vi "User Actor Core Init.vi"(0 "Module in":refnum<class "Module.lvclass">, 11 "Error in":errorcluster caption="Error in (no error)") -> (4 "Module out":refnum<class "Module.lvclass">, 15 "Error out":errorcluster)   [LabVIEW 2019, in "GP Module.lvlib" / "Module.lvclass"]
doc: "Initialize custom <B>Actor</B> resources. Typical actions:\n\n- Open/create own references.\n- Initialize SW resources.\n- Initialize HW resources.\n- Register additional user events. Beware that external user events are a potential for message racing as those are extra communication channels into <B>Actor</B> that does not follow the message order imposed by the Actor communication tree. If possible convert user event based APIs into message based APIs.\n\n<B>You should not invoke the Call Parent Method node when adding this override.</B>\n\nDefault action\n---------------\nNo action.\n\nSteen Schmidt\nGPower\n2/8 2017"
uses:
  Module.lvclass
  C:/Program Files (x86)/National Instruments/LabVIEW 2019/vi.lib/GPower/Actor/Library/Actor Class/Actor.lvclass
  <vilib>/GPower/Actor/Library/Actor Class/Actor.lvclass/Actor.ctl
  <vilib>/GPower/Actor/Library/Actor Interface Class/Actor Interface.lvclass/Actor Interface.ctl
  <vilib>/GPower/Actor/Library/Actor Class/Actor.lvclass
  <vilib>/GPower/UI/Library/GP UI.lvlib
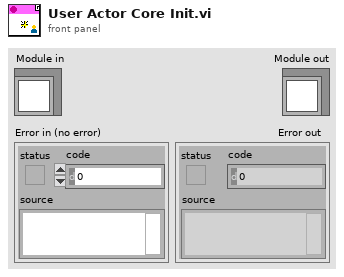
[diagram p1: front panel]
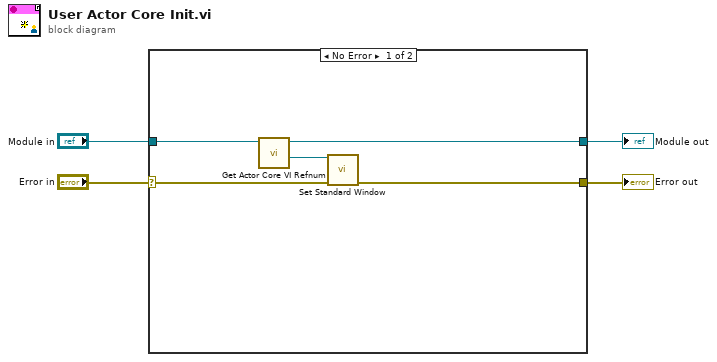
[diagram p0: block diagram]
diagram:
  n1 = case shown="No Error" "Error in" {
    selector: "Error in" -> [w7 w10]
    tunnel: "Module in" -> [w9 w11]
    tunnel: [w6 w10] -> w3
    tunnel: [w5 w11] -> w1
    frame No Error {
      n2 = call <vilib>:"Get Actor Core VI Refnum.vi"("Actor in"=w9) -> ("Actor Core VI Refnum"=w8:refnum<vi>, "Actor out"=w5:refnum<class "Module.lvclass">)  [unwired: 9 in]
      n3 = call <vilib>:"Set Standard Window.vi"("VI Refnum"=w8, "Error in"=w7) -> ("Error out"=w6:errorcluster)  [unwired: 13 in]
    }
    frame Error {
    }
  }
  "Module out" <- w1
  "Error out" <- w3
